vi "check network stream for data.vi"(7 "Queues in":T2, 11 "dataStream":T1) -> ()   [LabVIEW 2018]
uses:
  type defs/Queues.ctl
  type defs/data stream data.ctl
  supporting VIs/polymorphic VIs/enqueue for data processor.vi
  supporting VIs/polymorphic VIs/enqueue for file IO.vi
  supporting VIs/polymorphic VIs/enqueue for custom.vi
  <resource>/objmgr/ni.dex.rc
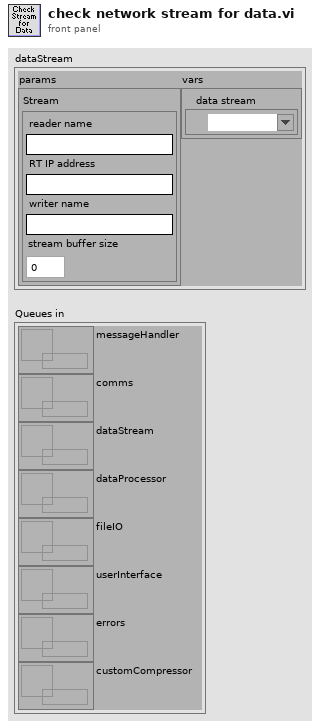
[diagram p1: front panel]
types:
  T1 = typedef "data stream data.ctl" = cluster{"params":cluster{"Stream":cluster{"reader name":string, "RT IP address":string, "writer name":string, "stream buffer size":i32}}, "vars":cluster{"data stream":refnum<k21>}}
  T2 = typedef "Queues.ctl" = cluster{"messageHandler":refnum<queue>, "comms":refnum<queue>, "dataStream":refnum<queue>, "dataProcessor":refnum<queue>, "fileIO":refnum<queue>, "userInterface":refnum<queue>, "errors":refnum<queue>, "customCompressor":refnum<queue>}
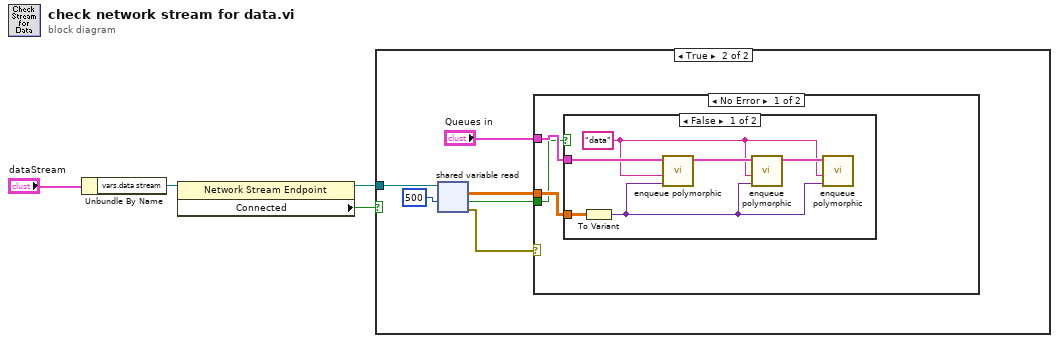
[diagram p0: block diagram]
diagram:
  n1 = Unbundle By Name("dataStream") -> ("vars.data stream"=w4:refnum<k21>)
  n2 = property class="Network Stream Endpoint"(reference=w4) -> (reference out=w2:refnum<k21>, "Connected"=w1:bool)  [unwired: 1 in, 1 out]
  n3 = case shown="True" w1 {
    tunnel: w2 -> [_ w6]
    frame False {
    }
    frame True {
      n4 = shared-variable-read(w6, 500 ("timeout ms (-1)")) -> (w5:errorcluster, w8:bool, w9:dbl[][])  [unwired: 1 in, 1 out]
      n5 = case shown="No Error" w5 {
        tunnel: "Queues in" -> [w13 _]
        tunnel: w9 -> [w12 _]
        tunnel: w8 -> [w11 _]
        frame No Error {
          n6 = case shown="False" w11 {
            tunnel: w12 -> [w18 _]
            tunnel: w13 -> [w19 _]
            frame False {
              w15 = "data" ("message")
              n7 = To Variant(anything=w18) -> (Variant=w14:variant)
              n8 = call-poly "enqueue polymorphic.vi"("data"=w14, "message"=w15, "Queues"=w19) -> ("Queues out"=w17:T2)  [unwired: 8 in]
              n9 = call-poly "enqueue polymorphic.vi"("data"=w14, "message"=w15, "Queues"=w17) -> ("Queues out"=w16:T2)  [unwired: 8 in]
              n10 = call-poly "enqueue polymorphic.vi"("data"=w14, "message"=w15, "Queues"=w16) -> ()  [unwired: 8 in, 1 out]
            }
            frame True {
            }
          }
        }
        frame Error {
        }
      }
    }
  }
